vi "Lockin Controller Only GPIB.vi"() -> ()   [LabVIEW 2013]
panel:
  in  "Tab Control":enum32{"Controls", "Error Codes"}(tab)
  in  "Input Configuration":u16(ring) items=["A", "A-B", "1 MOhm", "10 MOhm"]
  in  "Sensitivity":u16(ring) items=["2 nV/fA", "5 nV/fA", "10 nV/fA", "20 nV/fA", "50 nV/fA", "100 nV/fA", "200 nV/fA", "500 nV/fA", "1 uV/pA", "2 uV/pA", "5 uV/pA", "10 uV/pA", "20 uV/pA", "50 uV/pA", "100 uV/pA", "200 uV/pA", "500 uV/pA", "1 mV/nA", "2 mV/nA", "5 mV/nA", "10 mV/nA", "20 mV/nA", "50 mV/nA", "100 mV/nA", "200 mV/nA", "500 mV/nA", "1 V/uA"]
  in  "Time Constant":u16(ring) items=["10 us", "30 us", "100 us", "300 us", "1 ms", "3 ms", "10 ms", "30 ms", "100 ms", "300 ms", "1 s", "3 s", "10 s", "30 s", "100 s", "300 s", "1 ks", "3 ks", "10 ks", "30 ks"]
  out "Sensitivity Compensation":dbl
  in  "Stop Button":bool
  in  "Autophase":bool
  in  "Lockin GPIB Address":string="6"
  in  "Lockin  error out":errorcluster
  out "Digital Output":string="1.55532e-007\r"
  out "Lockin Output":dbl(knob) scale=-5.0..5.0
  # "Lockin Output Panel"
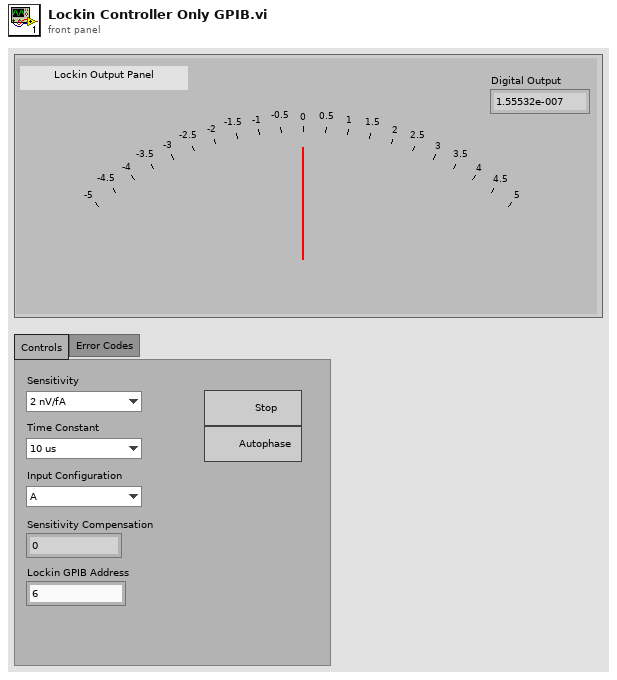
[diagram p1: front panel]
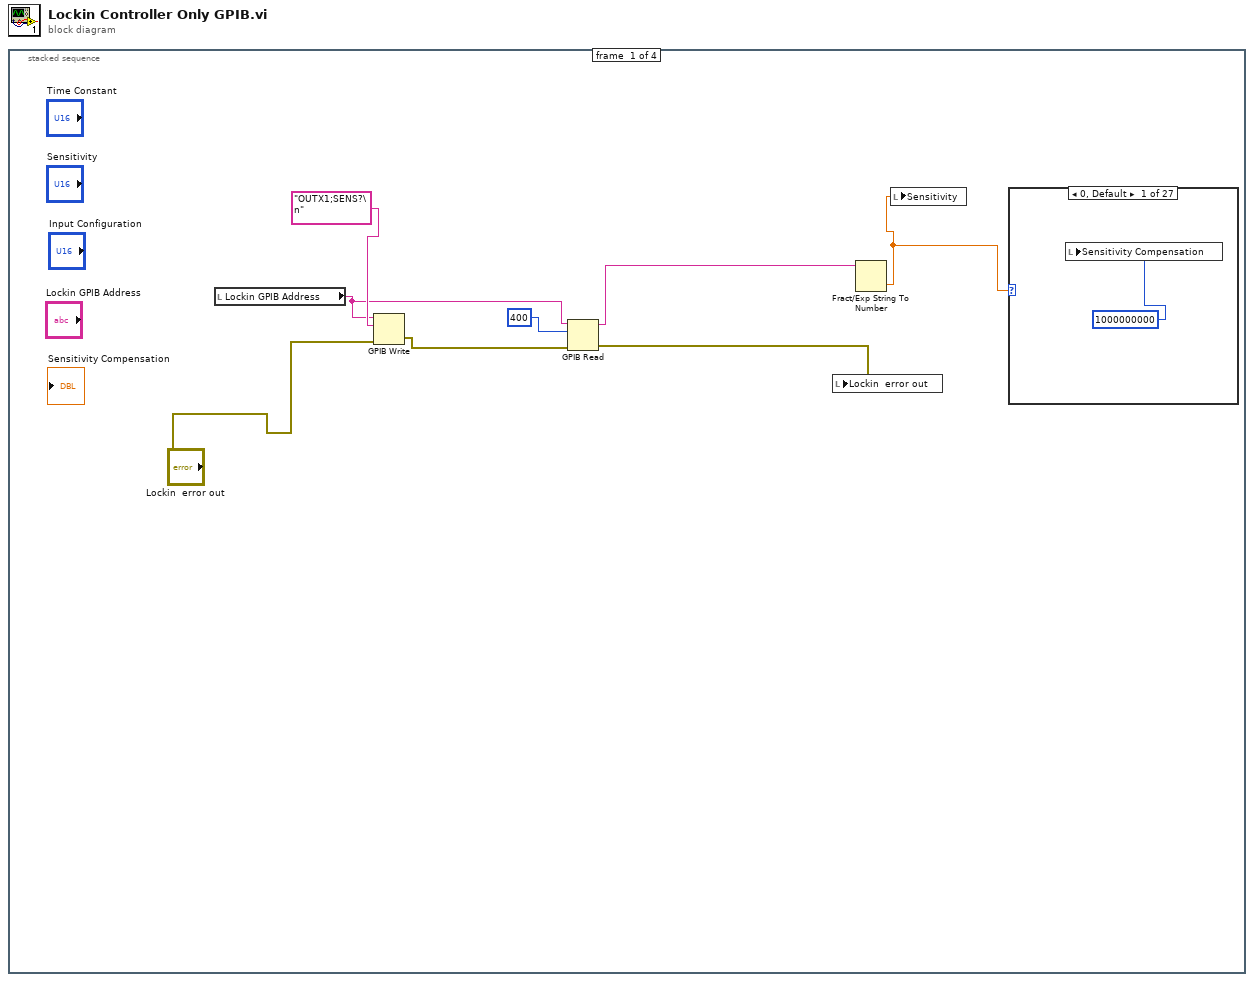
[diagram p0: block diagram]
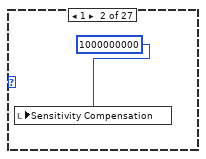
[diagram p2: hidden frame]
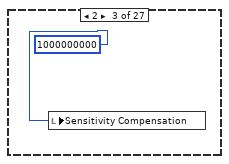
[diagram p3: hidden frame]
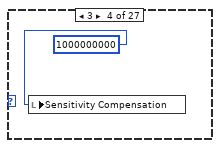
[diagram p4: hidden frame]
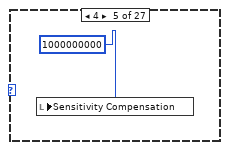
[diagram p5: hidden frame]
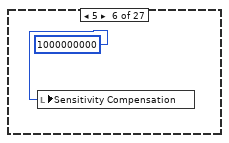
[diagram p6: hidden frame]
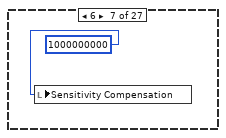
[diagram p7: hidden frame]
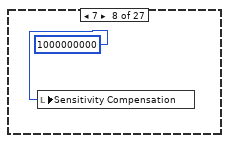
[diagram p8: hidden frame]
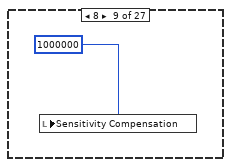
[diagram p9: hidden frame]
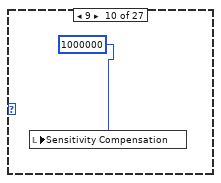
[diagram p10: hidden frame]
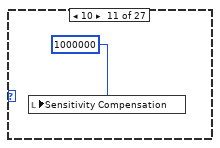
[diagram p11: hidden frame]
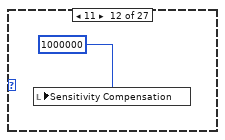
[diagram p12: hidden frame]
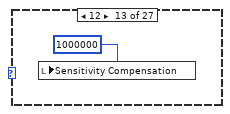
[diagram p13: hidden frame]
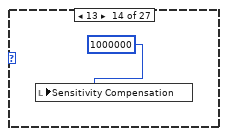
[diagram p14: hidden frame]
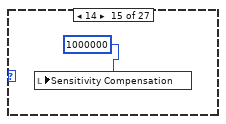
[diagram p15: hidden frame]
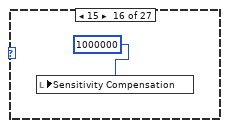
[diagram p16: hidden frame]
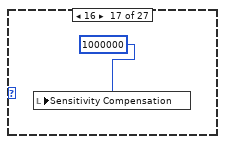
[diagram p17: hidden frame]
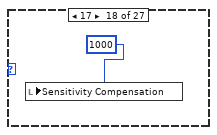
[diagram p18: hidden frame]
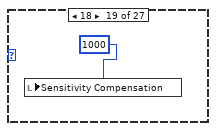
[diagram p19: hidden frame]
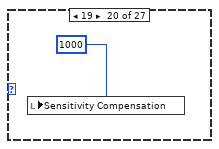
[diagram p20: hidden frame]
diagram:
  n1 = stacked-sequence {
    frame #0 {
      n2 = local read "Lockin GPIB Address"() -> (w3:string)
      n3 = GPIB Write(0:w3, 1:"OUTX1;SENS?\n", 3:"Lockin  error out") -> (6:w5:errorcluster)  [unwired: 2 in, 1 out]
      n4 = GPIB Read(0:w3, 1:400, 3:w5) -> (5:w2:string, 7:w4:errorcluster)  [unwired: 2 in, 1 out]
      n5 = local write "Lockin  error out"(w4) -> ()
      n6 = Fract/Exp String To Number(string=w2) -> (number=w8:dbl)  [unwired: 3 in, 1 out]
      n7 = local write "Sensitivity"(w8) -> ()
      n8 = case shown="0, Default" w8 {
        frame 0, Default {
          n9 = local write "Sensitivity Compensation"(1000000000) -> ()
        }
        frame 1 {
          n10 = local write "Sensitivity Compensation"(1000000000) -> ()
        }
        frame 2 {
          n11 = local write "Sensitivity Compensation"(1000000000) -> ()
        }
        frame 3 {
          n12 = local write "Sensitivity Compensation"(1000000000) -> ()
        }
        frame 4 {
          n13 = local write "Sensitivity Compensation"(1000000000) -> ()
        }
        frame 5 {
          n14 = local write "Sensitivity Compensation"(1000000000) -> ()
        }
        frame 6 {
          n15 = local write "Sensitivity Compensation"(1000000000) -> ()
        }
        frame 7 {
          n16 = local write "Sensitivity Compensation"(1000000000) -> ()
        }
        frame 8 {
          n17 = local write "Sensitivity Compensation"(1000000) -> ()
        }
        frame 9 {
          n18 = local write "Sensitivity Compensation"(1000000) -> ()
        }
        frame 10 {
          n19 = local write "Sensitivity Compensation"(1000000) -> ()
        }
        frame 11 {
          n20 = local write "Sensitivity Compensation"(1000000) -> ()
        }
        frame 12 {
          n21 = local write "Sensitivity Compensation"(1000000) -> ()
        }
        frame 13 {
          n22 = local write "Sensitivity Compensation"(1000000) -> ()
        }
        frame 14 {
          n23 = local write "Sensitivity Compensation"(1000000) -> ()
        }
        frame 15 {
          n24 = local write "Sensitivity Compensation"(1000000) -> ()
        }
        frame 16 {
          n25 = local write "Sensitivity Compensation"(1000000) -> ()
        }
        frame 17 {
          n26 = local write "Sensitivity Compensation"(1000) -> ()
        }
        frame 18 {
          n27 = local write "Sensitivity Compensation"(1000) -> ()
        }
        frame 19 {
          n28 = local write "Sensitivity Compensation"(1000) -> ()
        }
        frame 20 {
          n29 = local write "Sensitivity Compensation"(1000) -> ()
        }
        frame 21 {
          n30 = local write "Sensitivity Compensation"(1000) -> ()
        }
        frame 22 {
          n31 = local write "Sensitivity Compensation"(1000) -> ()
        }
        frame 23 {
          n32 = local write "Sensitivity Compensation"(1000) -> ()
        }
        frame 24 {
          n33 = local write "Sensitivity Compensation"(1000) -> ()
        }
        frame 25 {
          n34 = local write "Sensitivity Compensation"(1000) -> ()
        }
        frame 26 {
          n35 = local write "Sensitivity Compensation"(1) -> ()
        }
      }
    }
    frame #1 {
      n36 = local read "Lockin  error out"() -> (w39:errorcluster)
      n37 = local read "Lockin GPIB Address"() -> (w36:string)
      n38 = GPIB Write(0:w36, 1:"OUTX1;ISRC?\n", 3:w39) -> (6:w42:errorcluster)  [unwired: 2 in, 1 out]
      n39 = GPIB Read(0:w36, 1:400, 3:w42) -> (5:w37:string, 7:w40:errorcluster)  [unwired: 2 in, 1 out]
      n40 = Fract/Exp String To Number(string=w37) -> (number=w43:dbl)  [unwired: 3 in, 1 out]
      n41 = local write "Input Configuration"(w43) -> ()
      n42 = local write "Lockin  error out"(w40) -> ()
    }
    frame #2 {
      n43 = local read "Lockin  error out"() -> (w47:errorcluster)
      n44 = local read "Lockin GPIB Address"() -> (w44:string)
      n45 = GPIB Write(0:w44, 1:"OUTX1;OFLT?\n", 3:w47) -> (6:w50:errorcluster)  [unwired: 2 in, 1 out]
      n46 = GPIB Read(0:w44, 1:400, 3:w50) -> (5:w45:string, 7:w46:errorcluster)  [unwired: 2 in, 1 out]
      n47 = local write "Lockin  error out"(w46) -> ()
      n48 = Fract/Exp String To Number(string=w45) -> (number=w51:dbl)  [unwired: 3 in, 1 out]
      n49 = local write "Time Constant"(w51) -> ()
    }
    frame #3 {
      n50 = local read "Input Configuration"() -> (w54:u16)
      n51 = local read "Time Constant"() -> (w52:u16)
      n52 = local read "Sensitivity"() -> (w53:u16)
      n53 = while {
        shift-right: [w56] -> _
        shift-left: w54 -> [w61]
        shift-right: [w58] -> _
        shift-left: w53 -> [w60]
        shift-right: [w57] -> _
        shift-left: w52 -> [w59]
        stop <- "Stop Button" stop-if-true
        n54 = stacked-sequence {
          tunnel: w61 -> [w71 _ _ _]
          tunnel: w60 -> [_ _ w96 _]
          tunnel: w59 -> [_ w84 _ _]
          tunnel: [_ _ w94 _] -> w58
          tunnel: [_ w81 _ _] -> w57
          tunnel: [w68 _ _ _] -> w56
          frame #0 {
            n55 = local read "Input Configuration"() -> (w70:u16)
            n56 = Not Equal?(x=w70, y=w71) -> (x != y?=w69:bool)
            n57 = case shown="True" w69 {
              tunnel: [w72 w80] -> w68
              frame False {
                n58 = local read "Input Configuration"() -> (w72:u16)
              }
              frame True {
                n59 = local read "Lockin  error out"() -> (w76:errorcluster)
                n60 = local read "Lockin GPIB Address"() -> (w73:string)
                n61 = local read "Input Configuration"() -> (w80:u16)
                n62 = Number To Decimal String(number=w80) -> (decimal integer string=w78:string)  [unwired: 1 in]
                n63 = Concatenate Strings("ISRC", w78, "\r") -> (w74:string)
                n64 = GPIB Write(0:w73, 1:w74, 3:w76) -> (6:w75:errorcluster)  [unwired: 2 in, 1 out]
                n65 = local write "Lockin  error out"(w75) -> ()
              }
            }
          }
          frame #1 {
            n66 = local read "Time Constant"() -> (w83:u16)
            n67 = Not Equal?(x=w83, y=w84) -> (x != y?=w82:bool)
            n68 = case shown="True" w82 {
              tunnel: [w85 w90] -> w81
              frame False {
                n69 = local read "Time Constant"() -> (w85:u16)
              }
              frame True {
                n70 = local read "Lockin GPIB Address"() -> (w89:string)
                n71 = local read "Lockin  error out"() -> (w88:errorcluster)
                n72 = local read "Time Constant"() -> (w90:u16)
                n73 = Number To Decimal String(number=w90) -> (decimal integer string=w93:string)  [unwired: 1 in]
                n74 = Concatenate Strings("OFLT", w93, "\r") -> (w86:string)
                n75 = GPIB Write(0:w89, 1:w86, 3:w88) -> (6:w87:errorcluster)  [unwired: 2 in, 1 out]
                n76 = local write "Lockin  error out"(w87) -> ()
              }
            }
          }
          frame #2 {
            n77 = local read "Sensitivity"() -> (w97:u16)
            n78 = Not Equal?(x=w97, y=w96) -> (x != y?=w95:bool)
            n79 = case shown="True" w95 {
              tunnel: [w98 w103] -> w94
              frame False {
                n80 = local read "Sensitivity"() -> (w98:u16)
              }
              frame True {
                n81 = local read "Sensitivity"() -> (w103:u16)
                n82 = local read "Lockin  error out"() -> (w100:errorcluster)
                n83 = local read "Lockin GPIB Address"() -> (w102:string)
                n84 = Number To Decimal String(number=w103) -> (decimal integer string=w106:string)  [unwired: 1 in]
                n85 = Concatenate Strings("SENS", w106, "\r") -> (w101:string)
                n86 = GPIB Write(0:w102, 1:w101, 3:w100) -> (6:w99:errorcluster)  [unwired: 2 in, 1 out]
                n87 = local write "Lockin  error out"(w99) -> ()
                n88 = case shown="0, Default" w103 {
                  frame 0, Default {
                    n89 = local write "Sensitivity Compensation"(1000000000) -> ()
                  }
                  frame 1 {
                    n90 = local write "Sensitivity Compensation"(1000000000) -> ()
                  }
                  frame 2 {
                    n91 = local write "Sensitivity Compensation"(1000000000) -> ()
                  }
                  frame 3 {
                    n92 = local write "Sensitivity Compensation"(1000000000) -> ()
                  }
                  frame 4 {
                    n93 = local write "Sensitivity Compensation"(1000000000) -> ()
                  }
                  frame 5 {
                    n94 = local write "Sensitivity Compensation"(1000000000) -> ()
                  }
                  frame 6 {
                    n95 = local write "Sensitivity Compensation"(1000000000) -> ()
                  }
                  frame 7 {
                    n96 = local write "Sensitivity Compensation"(1000000000) -> ()
                  }
                  frame 8 {
                    n97 = local write "Sensitivity Compensation"(1000000) -> ()
                  }
                  frame 9 {
                    n98 = local write "Sensitivity Compensation"(1000000) -> ()
                  }
                  frame 10 {
                    n99 = local write "Sensitivity Compensation"(1000000) -> ()
                  }
                  frame 11 {
                    n100 = local write "Sensitivity Compensation"(1000000) -> ()
                  }
                  frame 12 {
                    n101 = local write "Sensitivity Compensation"(1000000) -> ()
                  }
                  frame 13 {
                    n102 = local write "Sensitivity Compensation"(1000000) -> ()
                  }
                  frame 14 {
                    n103 = local write "Sensitivity Compensation"(1000000) -> ()
                  }
                  frame 15 {
                    n104 = local write "Sensitivity Compensation"(1000000) -> ()
                  }
                  frame 16 {
                    n105 = local write "Sensitivity Compensation"(1000000) -> ()
                  }
                  frame 17 {
                    n106 = local write "Sensitivity Compensation"(1000) -> ()
                  }
                  frame 18 {
                    n107 = local write "Sensitivity Compensation"(1000) -> ()
                  }
                  frame 19 {
                    n108 = local write "Sensitivity Compensation"(1000) -> ()
                  }
                  frame 20 {
                    n109 = local write "Sensitivity Compensation"(1000) -> ()
                  }
                  frame 21 {
                    n110 = local write "Sensitivity Compensation"(1000) -> ()
                  }
                  frame 22 {
                    n111 = local write "Sensitivity Compensation"(1000) -> ()
                  }
                  frame 23 {
                    n112 = local write "Sensitivity Compensation"(1000) -> ()
                  }
                  frame 24 {
                    n113 = local write "Sensitivity Compensation"(1000) -> ()
                  }
                  frame 25 {
                    n114 = local write "Sensitivity Compensation"(1000) -> ()
                  }
                  frame 26 {
                    n115 = local write "Sensitivity Compensation"(1) -> ()
                  }
                }
              }
            }
          }
          frame #3 {
            n116 = local read "Lockin GPIB Address"() -> (w136:string)
            n117 = local read "Lockin  error out"() -> (w138:errorcluster)
            n118 = GPIB Write(0:w136, 1:"OUTX1;OUTP?1\n" ("string to write"), 3:w138) -> (6:w137:errorcluster)  [unwired: 2 in, 1 out]
            n119 = GPIB Read(0:w136, 1:400, 3:w137) -> (5:w135:string, 7:w139:errorcluster)  [unwired: 2 in, 1 out]
            "Digital Output" <- w135
            n120 = local write "Lockin  error out"(w139) -> ()
            n121 = local read "Sensitivity Compensation"() -> (w142:dbl)
            n122 = Fract/Exp String To Number(string=w135) -> (number=w143:dbl)  [unwired: 3 in, 1 out]
            n123 = Multiply(x=w143, y=w142) -> (x*y=→"Lockin Output":dbl)
          }
        }
        n124 = case shown="True" "Autophase" {
          frame False {
          }
          frame True {
            n125 = flat-sequence {
              frame #0 {
                n126 = local read "Lockin GPIB Address"() -> (w63:string)
                n127 = local read "Lockin  error out"() -> (w66:errorcluster)
                n128 = GPIB Write(0:w63, 1:"APHS\n", 3:w66) -> (6:w65:errorcluster)  [unwired: 2 in, 1 out]
                n129 = local write "Lockin  error out"(w65) -> ()
              }
              frame #1 {
                n130 = local write "Autophase"(FALSE) -> ()
              }
            }
          }
        }
      }
    }
  }
